vi "ini_read_cplx_double_vector.vi"(7 "section":string, 8 "error in":errorcluster, 9 "default":cdb[](array[numeric]), 10 "key":string, 11 "refnum in":T1) -> (0 "error out":errorcluster, 1 "values":cdb[](array[numeric]), 2 "found?":bool, 3 "refnum out":T1)   [LabVIEW 2018]
uses:
  <vilib>/Utility/config.llb/Config Data RefNum.ctl
  <vilib>/Utility/config.llb/Read Key (String).vi
  <vilib>/Utility/config.llb/NI_LVConfig.lvlib
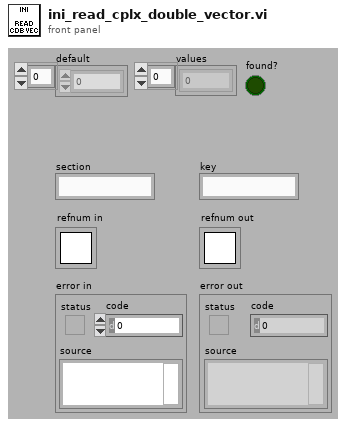
[diagram p1: front panel]
types:
  T1 = typedef "NI_LVConfig.lvlib/Config Data RefNum.ctl" = refnum<k1>
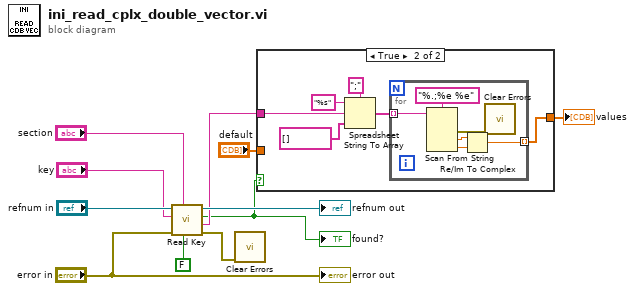
[diagram p0: block diagram]
diagram:
  n1 = call-poly <vilib>:"Read Key.vi"("read raw string? (F)"=FALSE, "section"="section", "error in (no error)"="error in", "key"="key", "refnum"="refnum in") -> ("error out"=w6:errorcluster, "value"=w5:string, "found?"=w4:bool, "refnum out"=→"refnum out":T1)  [unwired: 3 in]
  "found?" <- w4
  n2 = call <vilib>:"Clear Errors.vi"("error in (no error)"=w6) -> ()  [unwired: 5 in, 2 out]
  n3 = case shown="True" w4 {
    tunnel: w5 -> [_ w14]
    tunnel: "default" -> [w12 _]
    tunnel: [w12 w13] -> w2
    frame False {
    }
    frame True {
      n4 = Spreadsheet String To Array(delimiter (Tab)=";", format string="%s", spreadsheet string=w14, array type (2D Dbl)=string[] []) -> (array=w16:string[])
      n5 = for {
        tunnel: w16 -> [w24] mode=indexing
        tunnel: [w20] -> w13 mode=indexing
        n6 = Scan From String(format string="%.;%e %e", input string=w24) -> (error out=w19:errorcluster, output 1=w22:dbl, output 2=w21:dbl)  [unwired: 4 in, 2 out]
        n7 = Re/Im To Complex(1:w21, 2:w22) -> (0:w20:cdb)
        n8 = call <vilib>:"Clear Errors.vi"("error in (no error)"=w19) -> ()  [unwired: 5 in, 2 out]
      }
    }
  }
  "values" <- w2
  "error out" <- "error in"
